vi "CB PWM Command.vi"(8 "error in (no error)":errorcluster, 9 "Duty Cycle":i32 min=0 max=100, 10 "Leg":i32 min=0 max=6, 11 "VISA Refnum in":refnum<visa-resource-name>) -> (0 "error out":errorcluster, 2 "read buffer":string, 3 "VISA Refnum out":refnum<visa-resource-name>)   [LabVIEW 2022 SP3]
panel:
  out "return count":u32
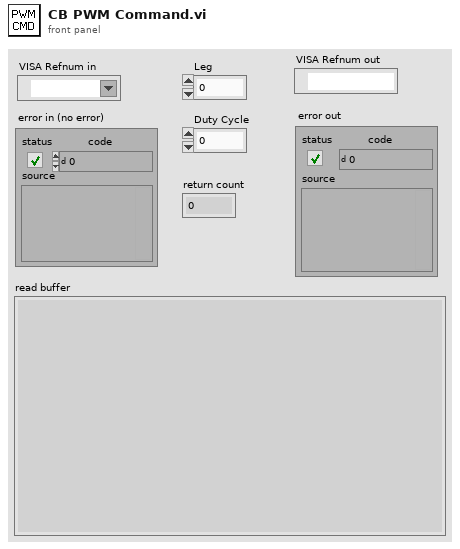
[diagram p1: front panel]
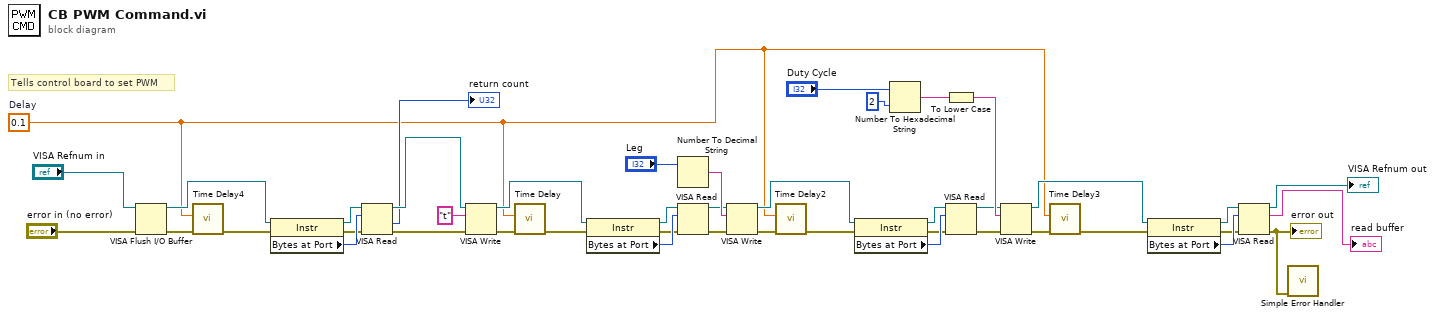
[diagram p0: block diagram]
diagram:
  w1 = 0.1  # Delay
  # "Tells control board to set PWM"
  n1 = VISA Flush I/O Buffer(VISA resource name="VISA Refnum in", error in (no error)="error in (no error)") -> (VISA resource name out=w6:refnum<visa-resource-name>, error out=w3:errorcluster)  [unwired: 1 in]
  n2 = call "Time Delay4"("error in (no error)"=w3, "Delay Time (s)"=w1) -> ("error out"=w2:errorcluster)  [unwired: 9 in]
  n3 = property class="Instr"(reference=w6, error in=w2) -> (reference out=w26:refnum<visa-resource-name>, error out=w8:errorcluster, "Bytes at Port"=w25:u32)
  n4 = VISA Read(VISA resource name=w26, byte count=w25, error in (no error)=w8) -> (VISA resource name out=w27:refnum<visa-resource-name>, return count=→"return count":u32, error out=w28:errorcluster)  [unwired: 1 out]
  n5 = VISA Write(VISA resource name=w27, write buffer="t", error in (no error)=w28) -> (VISA resource name out=w39:refnum<visa-resource-name>, error out=w44:errorcluster)  [unwired: 1 out]
  n6 = call "Time Delay"("error in (no error)"=w44, "Delay Time (s)"=w1) -> ("error out"=w24:errorcluster)  [unwired: 9 in]
  n7 = property class="Instr"(reference=w39, error in=w24) -> (reference out=w30:refnum<visa-resource-name>, error out=w23:errorcluster, "Bytes at Port"=w29:u32)
  n8 = Number To Decimal String(number="Leg") -> (decimal integer string=w33:string)  [unwired: 1 in]
  n9 = VISA Read(VISA resource name=w30, byte count=w29, error in (no error)=w23) -> (VISA resource name out=w32:refnum<visa-resource-name>, error out=w31:errorcluster)  [unwired: 2 out]
  n10 = VISA Write(VISA resource name=w32, write buffer=w33, error in (no error)=w31) -> (VISA resource name out=w38:refnum<visa-resource-name>, error out=w37:errorcluster)  [unwired: 1 out]
  n11 = call "Time Delay2"("error in (no error)"=w37, "Delay Time (s)"=w1) -> ("error out"=w18:errorcluster)  [unwired: 9 in]
  n12 = property class="Instr"(reference=w38, error in=w18) -> (reference out=w21:refnum<visa-resource-name>, error out=w19:errorcluster, "Bytes at Port"=w20:u32)
  n13 = Number To Hexadecimal String(1:i16 2 ("width (-)"), 2:"Duty Cycle") -> (0:w41:string)
  n14 = To Lower Case(string=w41) -> (all lower case string=w40:string)
  n15 = VISA Read(VISA resource name=w21, byte count=w20, error in (no error)=w19) -> (VISA resource name out=w22:refnum<visa-resource-name>, error out=w17:errorcluster)  [unwired: 2 out]
  n16 = VISA Write(VISA resource name=w22, write buffer=w40, error in (no error)=w17) -> (VISA resource name out=w42:refnum<visa-resource-name>, error out=w36:errorcluster)  [unwired: 1 out]
  n17 = call "Time Delay3"("error in (no error)"=w36, "Delay Time (s)"=w1) -> ("error out"=w12:errorcluster)  [unwired: 9 in]
  n18 = property class="Instr"(reference=w42, error in=w12) -> (reference out=w15:refnum<visa-resource-name>, error out=w11:errorcluster, "Bytes at Port"=w14:u32)
  n19 = VISA Read(VISA resource name=w15, byte count=w14, error in (no error)=w11) -> (VISA resource name out=→"VISA Refnum out":refnum<visa-resource-name>, read buffer=→"read buffer":string, error out=w9:errorcluster)  [unwired: 1 out]
  "error out" <- w9
  n20 = call <vilib>:"Simple Error Handler.vi"("error in (no error)"=w9) -> ()  [unwired: 4 in, 5 out]
